vi "timerInitialization.vi"(8 "error in (no error)":errorcluster, 11 "SpectrographHeartbeat in":refnum<class "SpectrographHeartbeat.lvclass">) -> (0 "error out":errorcluster, 3 "SpectrographHeartbeat out":refnum<class "SpectrographHeartbeat.lvclass">)   [LabVIEW 2016, in "SpectrographHeartbeat.lvclass"]
uses:
  SpectrographHeartbeat.lvclass
  SpectrographHeartbeat.lvclass/SpectrographHeartbeat.ctl
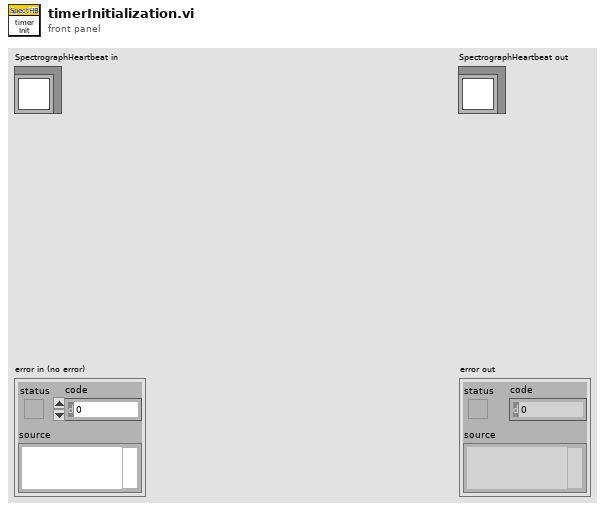
[diagram p1: front panel]
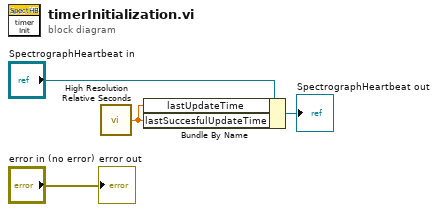
[diagram p0: block diagram]
diagram:
  n1 = call <vilib>:"High Resolution Relative Seconds.vi"() -> ("relative seconds"=w3:dbl)
  n2 = Bundle By Name(cluster="SpectrographHeartbeat in", "lastUpdateTime"=w3, "lastSuccesfulUpdateTime"=w3) -> (→"SpectrographHeartbeat out":refnum<class "SpectrographHeartbeat.lvclass">)
  "error out" <- "error in (no error)"
